vi "ql2proto_response_type_decode.vi"(11 "id":u32) -> (3 "response_type":T1)   [LabVIEW 2017]
uses:
  ql2proto_response_type.ctl
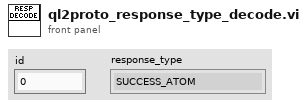
[diagram p1: front panel]
types:
  T1 = typedef "ql2proto_response_type.ctl" = enum8{"SUCCESS_ATOM", "SUCCESS_SEQUENCE", "SUCCESS_PARTIAL", "WAIT_COMPLETE", "SERVER_INFO", "CLIENT_ERROR", "COMPILE_ERROR", "RUNTIME_ERROR", "invalid"}
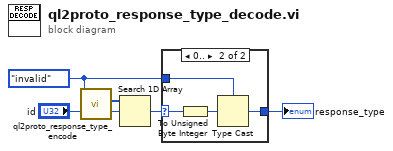
[diagram p0: block diagram]
diagram:
  w2 = ql2proto_response_type."invalid" ("response_type")
  n1 = call "ql2proto_response_type_encode.vi"("response_type"=w2) -> ("query_type_ids"=w1:u32[])  [unwired: 9 in, 1 out]
  n2 = Search 1D Array(1D array=w1, element="id") -> (index of element=w4:i32)  [unwired: 1 in]
  n3 = case shown="0.." w4 {
    selector: w4 -> [_ w7]
    tunnel: [w6 w10] -> w3
    tunnel: w2 -> [w6 w9]
    frame ..-1 {
    }
    frame 0.. {
      n4 = To Unsigned Byte Integer(number=w7) -> (unsigned 8bit integer=w8:u8)
      n5 = Type Cast(type=w9, x=w8) -> (*(type *) &x=w10:T1)
    }
  }
  "response_type" <- w3
